vi "RemoveTopic.vi"(8 "error in (no error)":errorcluster, 10 "Topic Name":string, 11 "Message Broker in":refnum<class "Message Broker.lvclass">) -> (0 "error out":errorcluster, 2 "Found?":bool, 3 "Message Broker out":refnum<class "Message Broker.lvclass">)   [LabVIEW 2016, in "Stream Mediator.lvlib" / "Message Broker.lvclass"]
doc: "--\nCopyright © 2017 Composed SystemsI All rights reserved.\n\nAuthor: Jon McBee <jon.mcbee@composed.io>\n\nThis library is provided \"AS IS\" ,WITHOUT WARRANTIES OR\nCONDITIONS OF ANY KIND, either express or implied.\n\nComposed Systems -- composed.io\n\nStream 0.0.1.1\nJon McBee - Composed Systems\nCopyright (c) 2017, Composed Systems"
uses:
  <userlib>/Composed Systems/Stream/Mediator/Classes/Message Broker/Message Broker.lvclass
  <userlib>/Composed Systems/Stream/Mediator/Classes/Message Broker/Message Broker.lvclass/Message Broker.ctl
  <userlib>/Composed Systems/Stream/Mediator/Classes/Topic Actor Look Up Table/Topic Actor Look Up Table.lvclass
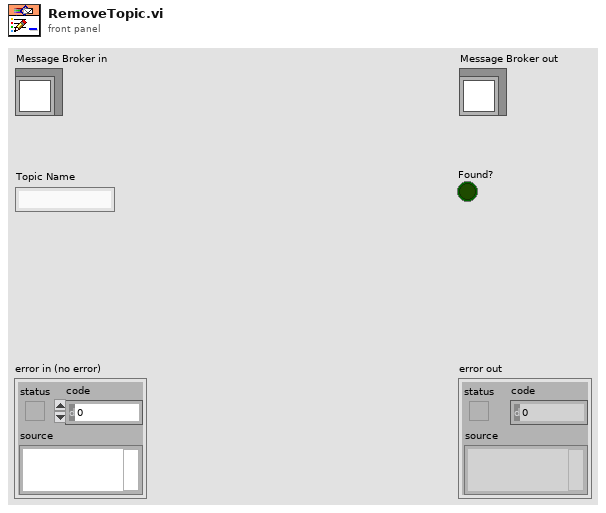
[diagram p1: front panel]
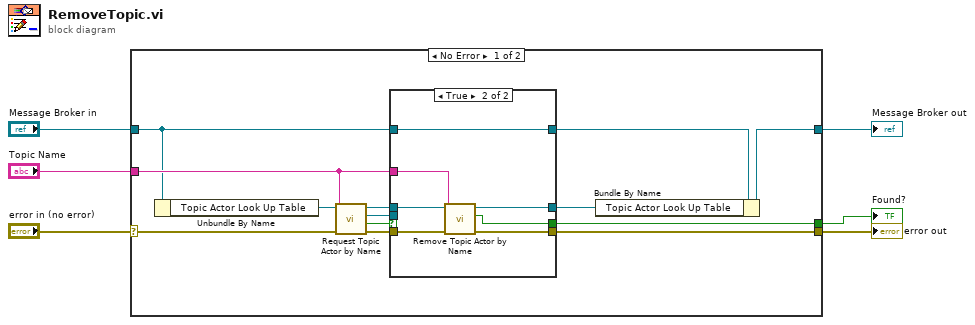
[diagram p0: block diagram]
diagram:
  n1 = case shown="No Error" "error in (no error)" {
    selector: "error in (no error)" -> [w12 w32]
    tunnel: [w19 w32] -> w5
    tunnel: [w17 w31] -> w3
    tunnel: "Message Broker in" -> [w11 w31]
    tunnel: "Topic Name" -> [w14 _]
    tunnel: [w7 _] -> w1
    frame No Error {
      n2 = Unbundle By Name(w11) -> ("Topic Actor Look Up Table"=w16:refnum<class "Topic Actor Look Up Table.lvclass">)
      n3 = call <userlib>:"Request Topic Actor by Name.vi"("error in (no error)"=w12, "Topic Actor"=w14, "Topic Actor Look Up Table in"=w16) -> ("error out"=w13:errorcluster, "Found?"=w9:bool, "Topic Actor Descriptor"=w8:refnum<class "Topic Actor Descriptor.lvclass">, "Topic Actor Look Up Table out"=w15:refnum<class "Topic Actor Look Up Table.lvclass">)  [unwired: 5 in]
      n4 = case shown="True" w9 {
        selector: w9 -> [w23 _]
        tunnel: [w20 w30] -> w19
        tunnel: [w21 w29] -> w18
        tunnel: w15 -> [w21 w25]
        tunnel: w14 -> [_ w28]
        tunnel: w13 -> [w20 w24]
        tunnel: [w22 w27] -> w10
        tunnel: w11 -> [w22 w27]
        tunnel: w8 -> [_ _]
        tunnel: [w23 w26] -> w7
        frame False {
        }
        frame True {
          n5 = call <userlib>:"Remove Topic Actor by Name.vi"("error in (no error)"=w24, "Topic Actor"=w28, "Topic Actor Look Up Table in"=w25) -> ("error out"=w30:errorcluster, "Found?"=w26:bool, "Topic Actor Look Up Table out"=w29:refnum<class "Topic Actor Look Up Table.lvclass">)  [unwired: 6 in]
        }
      }
      n6 = Bundle By Name(cluster=w10, "Topic Actor Look Up Table"=w18) -> (w17:refnum<class "Message Broker.lvclass">)
    }
    frame Error {
    }
  }
  "error out" <- w5
  "Message Broker out" <- w3
  "Found?" <- w1
